vi "Seek Audio File.vi"(8 "error in (no error)":errorcluster, 10 "Seek Position":u64, 11 "Audio File Refnum In":refnum<file>) -> (0 "error out":errorcluster, 3 "Audio File Refnum Out":refnum<file>)   [LabVIEW 2020, in "G-Audio.lvlib"]
doc: "Seek to the specified sample position. Subsequent audio file read will begin at this sample position."
uses:
  G-Audio.lvlib
  <vilib>/Utility/error.llb/Error Cluster From Error Code.vi
  lib/g_audio_x86.dll
  lib/g_audio_x64.dll
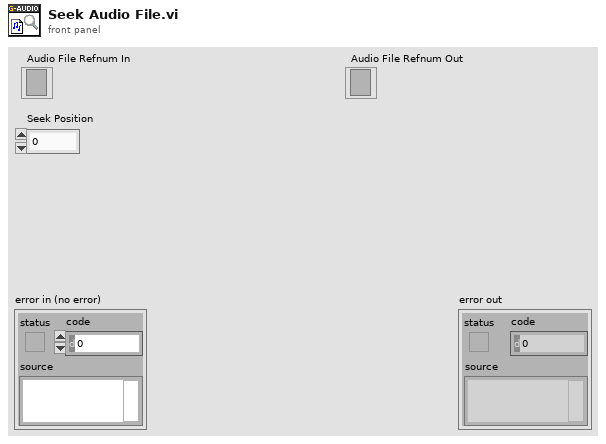
[diagram p1: front panel]
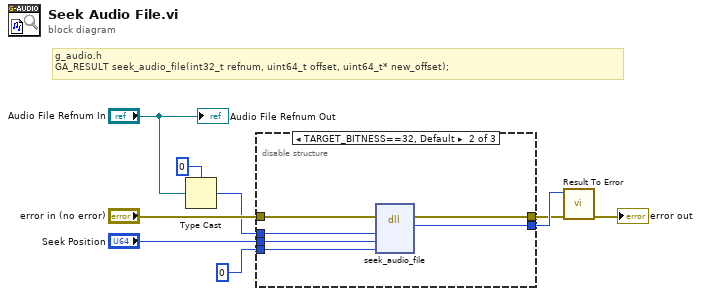
[diagram p0: block diagram]
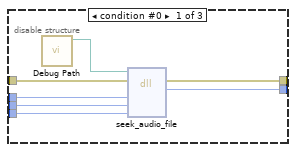
[diagram p2: hidden frame]
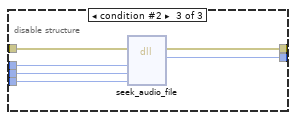
[diagram p3: hidden frame]
diagram:
  # "g_audio.h\nGA_RESULT seek_audio_file(int32_t refnum, uint64_t offset, uint64_t* new_offset);"
  n1 = Type Cast(type=0, x="Audio File Refnum In") -> (*(type *) &x=w6:i32)
  n2 = disable-structure shown="TARGET_BITNESS==32, Default" {
    disable-tunnel: "error in (no error)" -> [w16 w22 w28]
    disable-tunnel: [w14 w20 w26] -> w3
    disable-tunnel: [w15 w21 w27] -> w2
    disable-tunnel: "Seek Position" -> [w13 w19 w25]
    disable-tunnel: w6 -> [w12 w18 w24]
    disable-tunnel: u64 0 -> [w11 w17 w23]
    frame condition #0 {
      n3 = call "Debug Path.vi"() -> ("Debug Path"=w10:path)  [unwired: 11 in]
      n4 = dll-call lib="?" fn="seek_audio_file"(path in=w10, error in=w16, "refnum"=w12, "offset"=w13, "new_offset"=w11) -> (error out=w15:errorcluster, "result"=w14:i32)  [unwired: 4 in, 1 out]
    }
    frame condition #1 (active) {
      n5 = dll-call lib="C:/github/dataflowg/g-audio/src/LabVIEW/G-Audio/lib/g_audio_x86.*" fn="seek_audio_file"(error in=w22, "refnum"=w18, "offset"=w19, "new_offset"=w17) -> (error out=w21:errorcluster, "result"=w20:i32)  [unwired: 5 in, 1 out]
    }
    frame condition #2 {
      n6 = dll-call lib="C:/github/dataflowg/g-audio/src/LabVIEW/G-Audio/lib/g_audio_x64.*" fn="seek_audio_file"(error in=w28, "refnum"=w24, "offset"=w25, "new_offset"=w23) -> (error out=w27:errorcluster, "result"=w26:i32)  [unwired: 5 in, 1 out]
    }
  }
  n7 = call "Result To Error.vi"("error in (no error)"=w2, "Result Code"=w3) -> ("error out"=→"error out":errorcluster)  [unwired: 9 in]
  "Audio File Refnum Out" <- "Audio File Refnum In"
